vi "CreatingandAccessingFile2s.vi"() -> ()   [LabVIEW 2020]
panel:
  in  "count":i32
  out "text":string
  in  "file path (use dialog)":path
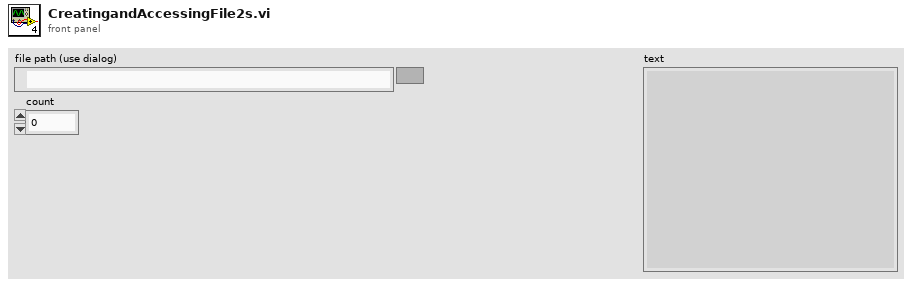
[diagram p1: front panel]
types:
  T1 = enum16{"open", "replace", "create", "open or create", "replace or create", "replace or create with confirmation"}
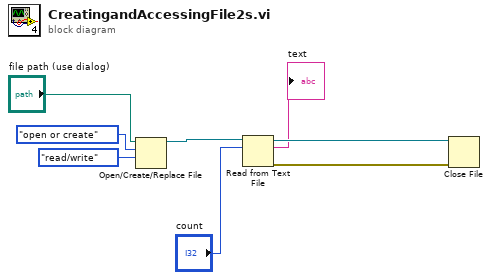
[diagram p0: block diagram]
diagram:
  n1 = Open/Create/Replace File(file path (use dialog)="file path (use dialog)", operation (0:open)=T1."open or create", access (0:read/write)=enum16{"read/write", "read-only", "write-only"}."read/write") -> (refnum out=w3:refnum<file>)  [unwired: 3 in, 2 out]
  n2 = Read from Text File(file (use dialog)=w3, count="count") -> (refnum out=w5:refnum<file>, text=→"text":string, error out=w4:errorcluster)  [unwired: 2 in, 1 out]
  n3 = Close File(refnum=w5, error in=w4) -> ()  [unwired: 2 out]
